vi "OA Timebase Plot.vi"   [LabVIEW 2017]
doc: "Draws a timebase plot with unfiltered or filtered data on an XY graph. The unfiltered data comes from the <B>even-angle signals</B> input, the filtered data from the <B>magnitudes</B> and <B>phases [phase lag]</B> inputs. The timebase plot displays the amplitude of a signal as a function of time and marks the tachometer trigger point on the plot. The data type you wire to the <B>even-angle signals</B> input determines the polymorphic instance to use."
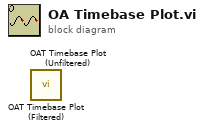
[diagram p0: block diagram]
diagram:
  n1 = call <vilib>:"OAT Timebase Plot (Filtered).vi"() -> ()  [unwired: 13 in, 3 out]
  n2 = call <vilib>:"OAT Timebase Plot (Unfiltered).vi"() -> ()  [unwired: 13 in, 3 out]
